vi "qHIB.vi"(0 "System no.":i32=1 min=1 max=4 step=1, 1 "DeviceID":i32[](array[numeric]), 2 "DeviceButton":i32[](array[numeric]), 3 "All DeviceIDs?":bool, 5 "error in":errorcluster) -> (14 "State":i32[](array[numeric]), 19 "error out":errorcluster)   [LabVIEW 2026]
doc: "Returns the state of the buttons of a Human Interface Device (HID). See controller user manual for details.\n\nC-867: \n\nF-206, M-8X0: Only for GCS syntax version = GCS 2.0 or higher (Check with CSV?.vi. If CSV?.vi is not supported, syntax version is GCS 1.0)."
panel:
  # "Returns the state of the buttons of a Human Interface Device (HID)."
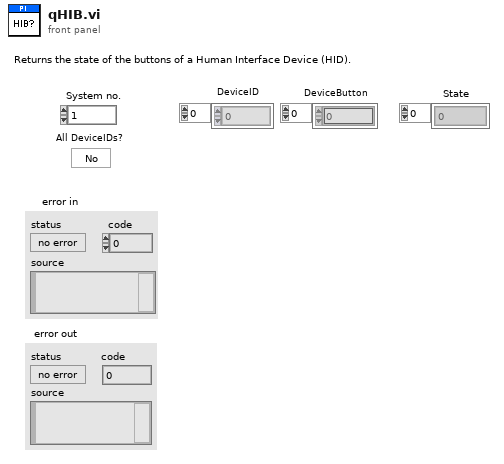
[diagram p1: front panel]
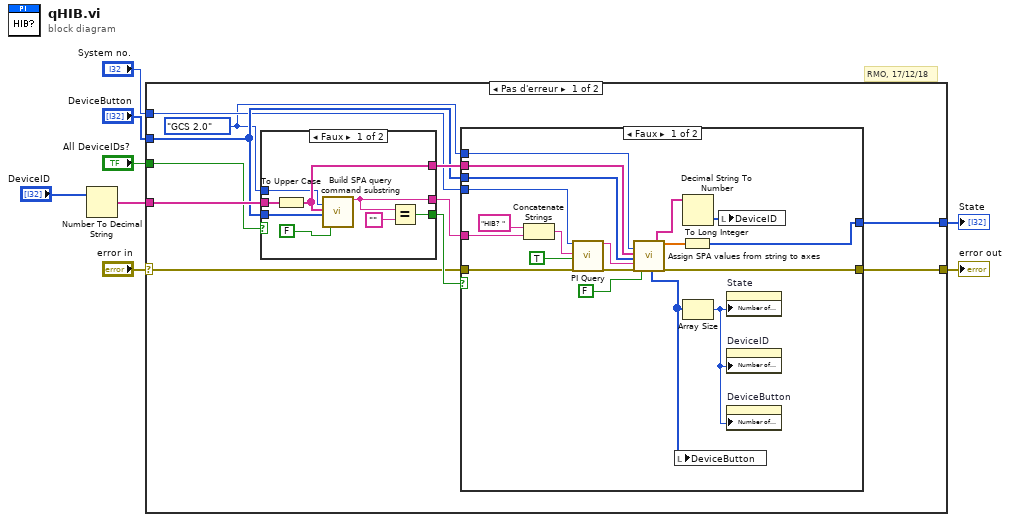
[diagram p0: block diagram]
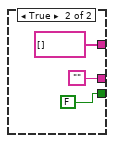
[diagram p2: hidden frame]
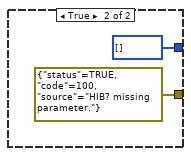
[diagram p3: hidden frame]
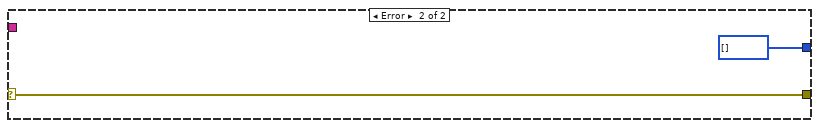
[diagram p4: hidden frame]
diagram:
  # "RMO, 17/12/18"
  n1 = Number To Decimal String(number="DeviceID") -> (decimal integer string=w3:string[])  [unwired: 1 out]
  n2 = case shown="Pas d'erreur" "error in" {
    selector: "error in" -> [w9 w52]
    tunnel: w3 -> [w19 _]
    tunnel: "System no." -> [w11 _]
    tunnel: "DeviceButton" -> [w16 _]
    tunnel: [w15 w52] -> w6
    tunnel: [w13 i32[] []] -> w5
    tunnel: "All DeviceIDs?" -> [w12 _]
    frame No Error {
      w10 = enum16{"GCS 1.0", "GCS 2.0"}."GCS 2.0" ("Syntax")
      n3 = case shown="Faux" w12 {
        tunnel: w19 -> [w27 _]
        tunnel: [w26 "" ("Command substring")] -> w18
        tunnel: [w25 string[] [] ("Designator to query")] -> w17
        tunnel: w16 -> [w24 _]
        tunnel: [w23 FALSE] -> w14
        tunnel: w10 -> [w22 _]
        frame False {
          n4 = To Upper Case(1:w27) -> (0:w25:string[])
          n5 = call "Build SPA query command substring.vi"("Syntax"=w22, "Axes to query"=w25, "Parameter number"=w24, "Parameter no. format \n(Decimal: FALSE)"=FALSE ("Parameter no. format \n(Decimal: FALSE)")) -> ("Command substring"=w26:string)  [unwired: 3 in, 12 out]
          n6 = Equal?(x=w26, y="" ("x")) -> (x = y?=w23:bool)
        }
        frame True {
        }
      }
      n7 = case shown="Faux" w14 {
        tunnel: w9 -> [w43 _]
        tunnel: w18 -> [w46 _]
        tunnel: w17 -> [w45 _]
        tunnel: w11 -> [w42 _]
        tunnel: w16 -> [w44 _]
        tunnel: [w39 errorcluster {"status"=TRUE, "code"=100, "source"="HIB? missing parameter."} ("error out")] -> w15
        tunnel: [w33 i32[] []] -> w13
        tunnel: w10 -> [w41 _]
        frame False {
          n8 = Concatenate Strings("HIB? ", w46) -> (w47:string)
          n9 = call "PI Query.vi"("System no."=w42, "String to send"=w47, "Attach termination char.?"=TRUE ("Attach Linefeed?"), "error in"=w43) -> ("String read"=w31:string, "error out"=w32:errorcluster)  [unwired: 3 in, 11 out]
          n10 = call "Assign SPA values from string to axes.vi"("Syntax"=w41, "Queried axes"=w45, "Parameter no."=w44, "Input string"=w31, "error in"=w32, "Parameter no. format \n(Decimal: FALSE)"=FALSE ("Parameter no. format \n(Decimal: FALSE)")) -> ("Parameter no. out"=w38:i32[], "Queried axes out"=w37:string[], "Parameter values"=w34:dbl[], "error out"=w39:errorcluster)  [unwired: 2 in, 8 out]
          n11 = local write "DeviceButton"(w38) -> ()
          n12 = To Long Integer(number=w34) -> (32bit integer=w33:i32[])
          n13 = Decimal String To Number(string=w37) -> (number=w36:i32[])  [unwired: 3 out]
          n14 = Array Size(array=w38) -> (size(s)=w35:i32)
          n15 = local write "DeviceID"(w36) -> ()
          n16 = property on="State" class="Tabl (strict)"("Number of Rows"=w35) -> ()  [unwired: 2 in, 2 out]
          n17 = property on="DeviceID" class="Tabl (strict)"("Number of Rows"=w35) -> ()  [unwired: 2 in, 2 out]
          n18 = property on="DeviceButton" class="Tabl (strict)"("Number of Rows"=w35) -> ()  [unwired: 2 in, 2 out]
        }
        frame True {
        }
      }
    }
    frame Error {
    }
  }
  "error out" <- w6
  "State" <- w5
